vi "Write I16.vi"(10 "I16":i16, 11 "Event in":refnum<class "Event I16.lvclass">) -> (3 "Event out":refnum<class "Event I16.lvclass">)   [LabVIEW 2016, in "Event Actors.lvlib" / "Event I16.lvclass"]
uses:
  Event I16.lvclass
  Event I16.lvclass/Event I16.ctl
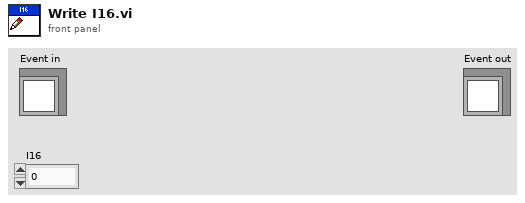
[diagram p1: front panel]
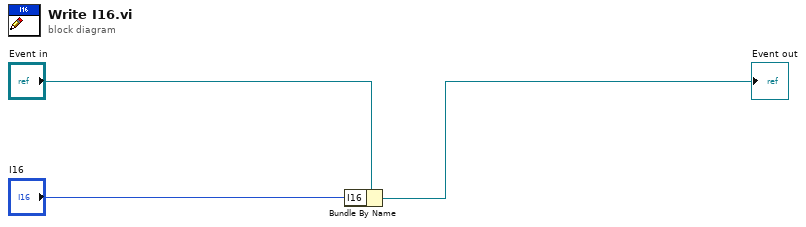
[diagram p0: block diagram]
diagram:
  n1 = Bundle By Name(cluster="Event in", "I16"="I16") -> (→"Event out":refnum<class "Event I16.lvclass">)
